vi "save data.vi"() -> ()   [LabVIEW 2014]
uses:
  <vilib>/Utility/file.llb/Write To Spreadsheet File (DBL).vi
panel:
  in  "Path":path
  in  "Acquisition time (s)":dbl
  in  "Period":dbl
  out "Waveform Graph":cluster{i32, "Period":dbl, i32[]}(graph)
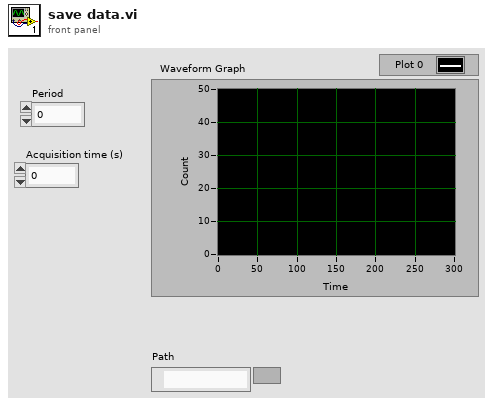
[diagram p1: front panel]
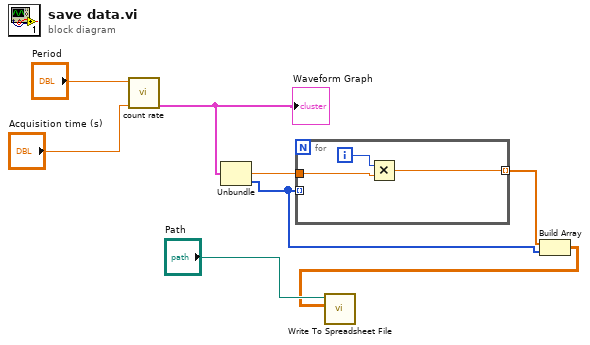
[diagram p0: block diagram]
diagram:
  n1 = call "count rate.vi"("Acquisition time (s)"="Acquisition time (s)", "Period"="Period") -> ("output cluster"=w5:cluster{i32, "Period":dbl, i32[]})  [unwired: 8 in, 1 out]
  "Waveform Graph" <- w5
  n2 = Unbundle(w5) -> ("Period"=w4:dbl, w2:i32[])  [unwired: 1 out]
  n3 = for {
    tunnel: w2 -> [_] mode=indexing
    tunnel: w4 -> [w10]
    tunnel: [w9] -> w3 mode=indexing
    i -> [w11]
    n4 = Multiply(x=w11, y=w10) -> (x*y=w9:dbl)
  }
  n5 = Build Array(w3, w2) -> (w1:dbl[][])
  n6 = call-poly <vilib>:"Write To Spreadsheet File.vi"("2D data"=w1, "file path (dialog if empty)"="Path") -> ()  [unwired: 6 in, 1 out]
